vi "CLC_Init.vi"(8 "error in (no error)":errorcluster, 11 "TCPIPin":T1={"address"="192.168.100.111", "remote port or service name"=5025, "timeout ms (60000)"=10000}) -> (0 "error out":errorcluster, 1 "Status":bool, 3 "TCPIPin 2":T1={"address"="192.168.100.111", "remote port or service name"=5025, "timeout ms (60000)"=10000})   [LabVIEW 2023]
panel:
  out "data out":string
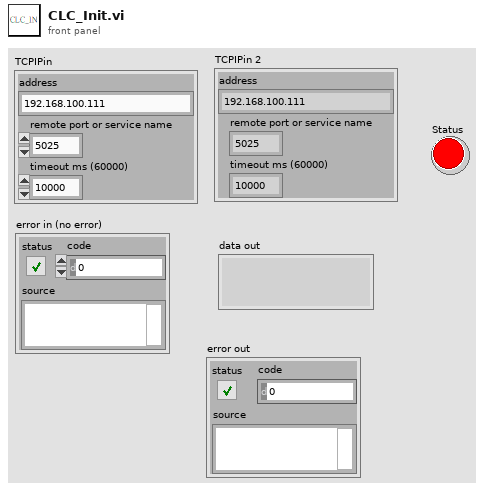
[diagram p1: front panel]
types:
  T1 = cluster{"address":string, "remote port or service name":u16, "timeout ms (60000)":i32}
  T2 = enum16{"Standard", "Buffered", "CRLF", "Immediate"}
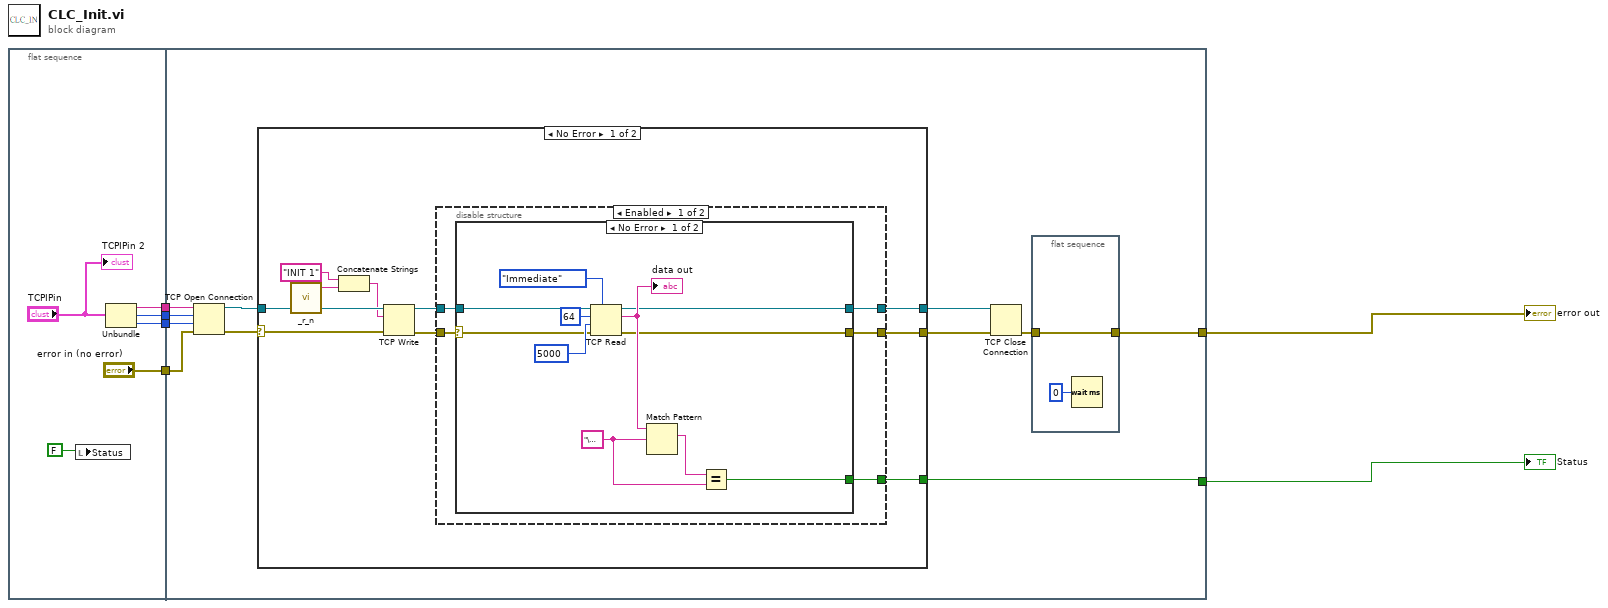
[diagram p0: block diagram]
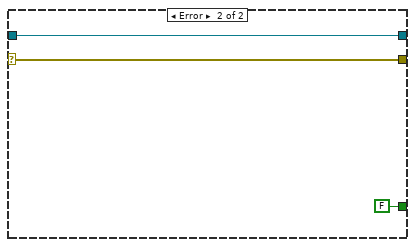
[diagram p2: hidden frame]
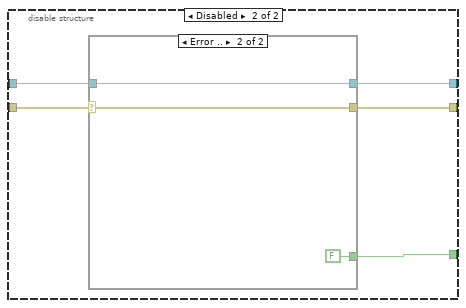
[diagram p3: hidden frame]
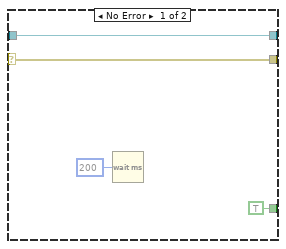
[diagram p4: hidden frame]
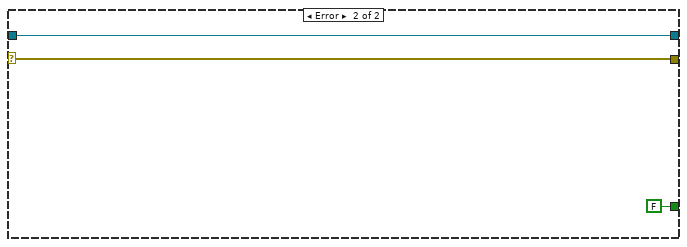
[diagram p5: hidden frame]
diagram:
  n1 = flat-sequence {
    tunnel: [w12] -> w6
    tunnel: [w11] -> w5
    tunnel: [w10] -> w4
    tunnel: ["error in (no error)"] -> w1
    tunnel: w6 -> [w19]
    tunnel: w5 -> [w17]
    tunnel: w4 -> [w20]
    tunnel: [w18] -> w3
    tunnel: [w16] -> w2
    tunnel: w1 -> [w13]
    frame #0 {
      n2 = local write "Status"(FALSE) -> ()
      n3 = Unbundle("TCPIPin") -> ("address"=w12:string, "remote port or service name"=w11:u16, "timeout ms (60000)"=w10:i32)
      "TCPIPin 2" <- "TCPIPin"
    }
    frame #1 {
      n4 = TCP Open Connection(address=w19, remote port or service name=w17, timeout ms (60000)=w20, error in (no error)=w13) -> (connection ID=w21:refnum<k5>, error out=w23:errorcluster)  [unwired: 1 in]
      n5 = case shown="No Error" w23 {
        selector: w23 -> [w32 w67]
        tunnel: w21 -> [w33 w66]
        tunnel: [w25 w67] -> w14
        tunnel: [w27 w66] -> w15
        tunnel: [w24 FALSE] -> w16
        frame No Error {
          n6 = call "_r_n.vi"() -> ("command"=w31:string)  [unwired: 5 in]
          n7 = Concatenate Strings("INIT 1" ("data in"), w31) -> (w29:string)
          n8 = TCP Write(connection ID=w33, data in=w29, error in (no error)=w32) -> (connection ID out=w28:refnum<k5>, error out=w26:errorcluster)  [unwired: 1 in, 1 out]
          n9 = disable-structure shown="Enabled" {
            disable-tunnel: [w38 w57] -> w24
            disable-tunnel: w26 -> [w34 w56]
            disable-tunnel: w28 -> [w37 w55]
            disable-tunnel: [w36 w54] -> w25
            disable-tunnel: [w35 w53] -> w27
            frame Enabled {
              n10 = case shown="No Error" w34 {
                selector: w34 -> [w39 w52]
                tunnel: [w43 FALSE] -> w38
                tunnel: w37 -> [w42 w51]
                tunnel: [w41 w52] -> w36
                tunnel: [w40 w51] -> w35
                frame No Error {
                  w44 = "\u0000" ("string")
                  n11 = TCP Read(connection ID=w42, bytes to read=64, error in (no error)=w39, 7:T2."Immediate" ("mode (standard)"), 9:5000 ("timeout ms (25000)")) -> (connection ID out=w40:refnum<k5>, data out=w46:string, error out=w41:errorcluster)
                  "data out" <- w46
                  n12 = Match Pattern(string=w46, regular expression=w44) -> (match substring=w45:string)  [unwired: 1 in, 3 out]
                  n13 = Equal?(x=w45, y=w44) -> (x = y?=w43:bool)
                }
                frame Error {
                }
              }
            }
            frame Disabled {
              n14 = case shown="Error .." w56 {
                selector: w56 -> [w59 w64]
                tunnel: [TRUE FALSE] -> w57
                tunnel: w55 -> [w58 w63]
                tunnel: [w59 w64] -> w54
                tunnel: [w58 w63] -> w53
                frame No Error {
                  n15 = Wait (ms)(milliseconds to wait=u32 200) -> ()  [unwired: 1 out]
                }
                frame Error {
                }
              }
            }
          }
        }
        frame Error {
        }
      }
      n16 = TCP Close Connection(connection ID=w15, error in (no error)=w14) -> (error out=w22:errorcluster)  [unwired: 1 in, 1 out]
      n17 = flat-sequence {
        tunnel: w22 -> [w69]
        tunnel: [w69] -> w18
        frame #0 {
          n18 = Wait (ms)(milliseconds to wait=u32 0) -> ()  [unwired: 1 out]
        }
      }
    }
  }
  "error out" <- w3
  "Status" <- w2
